vi "Close DI Ref.vi"(8 "error in (no error)":errorcluster, 11 "PXI 6515 in":refnum<class "PXI 6515.lvclass">) -> (0 "error out":errorcluster, 3 "PXI 6515 out":refnum<class "PXI 6515.lvclass">)   [LabVIEW 2016, in "DAQ IO.lvlib" / "PXI 6515.lvclass"]
uses:
  PXI 6515.lvclass
  PXI 6515.lvclass/PXI 6515.ctl
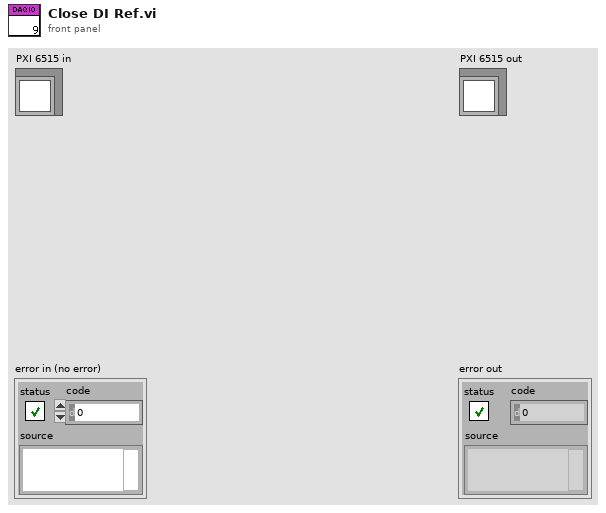
[diagram p1: front panel]
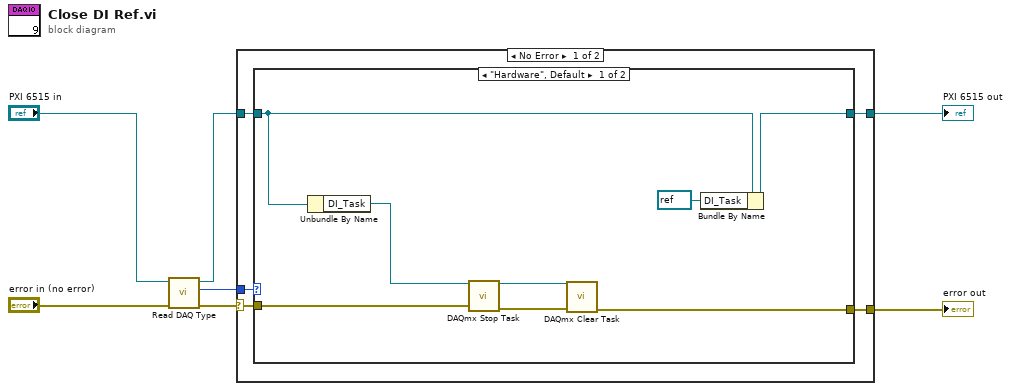
[diagram p0: block diagram]
diagram:
  n1 = call-dynamic "Read DAQ Type.vi"("error in (no error)"="error in (no error)", "PXI 6515 in"="PXI 6515 in") -> ("error out"=w6:errorcluster, "DAQ Type"=w5:enum16{"Hardware", "Simulation"}, "PXI 6515 out"=w1:refnum<class "PXI 6515.lvclass">)  [unwired: 7 in]
  n2 = case shown="No Error" w6 {
    selector: w6 -> [w12 w23]
    tunnel: w5 -> [w11 _]
    tunnel: w1 -> [w10 w24]
    tunnel: [w9 w24] -> w4
    tunnel: [w8 w23] -> w3
    frame No Error {
      n3 = case shown="\"Hardware\", Default" w11 {
        tunnel: w12 -> [w20 w21]
        tunnel: w10 -> [w16 w22]
        tunnel: [w14 w22] -> w9
        tunnel: [w15 w21] -> w8
        frame "Hardware", Default {
          n4 = Unbundle By Name(w16) -> ("DI_Task"=w18:refnum<k21>)
          n5 = call <vilib>:"DAQmx Stop Task.vi"("task/channels in"=w18, "error in"=w20) -> ("task out"=w17:refnum<k21>, "error out"=w19:errorcluster)  [unwired: 12 in]
          n6 = call <vilib>:"DAQmx Clear Task.vi"("task in"=w17, "error in"=w19) -> ("error out"=w15:errorcluster)  [unwired: 13 in]
          n7 = Bundle By Name(cluster=w16, "DI_Task"=refnum<k21> refnum) -> (w14:refnum<class "PXI 6515.lvclass">)
        }
        frame "Simulation" {
        }
      }
    }
    frame Error {
    }
  }
  "error out" <- w3
  "PXI 6515 out" <- w4
